vi "Post Upload.vi"() -> ()   [LabVIEW 2012]
uses:
  <vilib>/LVH/i3 Twitter/i3-twitter.lvlib
  <vilib>/LVH/i3 Twitter/SubVIs/Twitter Open - Desktop.vi
  <vilib>/LVH/i3 Twitter/Tweets with Media/Post Media Tweet - From File.vi
panel:
  out "resulting string":string
  out "file names":string[](array[string])
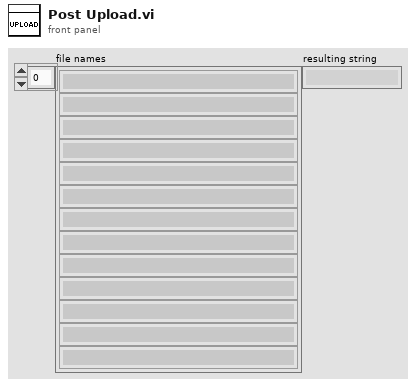
[diagram p1: front panel]
types:
  T1 = typedef "i3-twitter.lvlib/Twitter Handle.ctl" = cluster{"OAuth Credentials":T2, "since ID":string, "max ID":string, "Screen Name":string}
  T2 = typedef "i3-oauth.lvlib/OAuth Handle.ctl" = cluster{"Signature Method":T3, "Version":string, "Client":T4, "Access":T4}
  T3 = typedef "i3-oauth.lvlib/Signature Method.ctl" = enum16{"HMAC-MD5", "HMAC-SHA1", "HMAC-SHA224", "HMAC-SHA256", "HMAC-SHA384", "HMAC-SHA512"}
  T4 = typedef "i3-oauth.lvlib/Credentials.ctl" = cluster{"Token":string, "Secret":string}
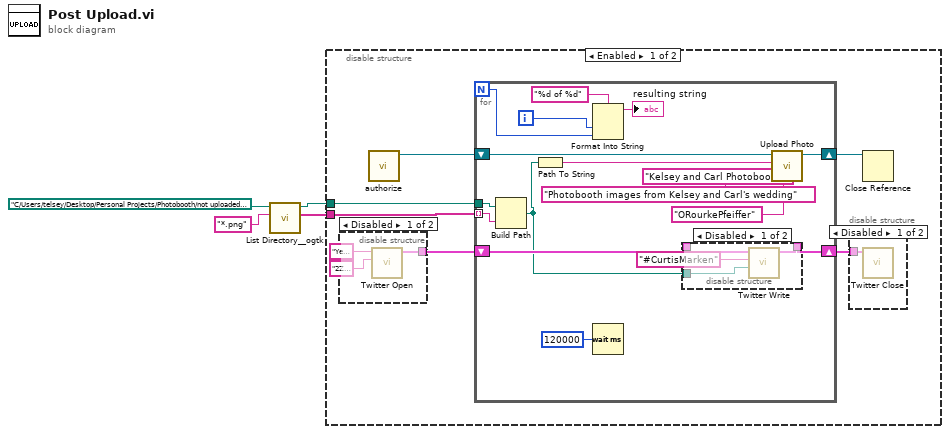
[diagram p0: block diagram]
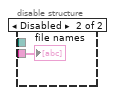
[diagram p5: hidden frame]
diagram:
  n1 = call <userlib>:"List Directory__ogtk.vi"("pattern"="*.png", "directory path"=path "C:/Users/telsey/Desktop/Personal Projects/Photobooth/not uploaded yet") -> ("file names"=w3:string[], "dup directory path"=w1:path)  [unwired: 2 in, 2 out]
  n2 = disable-structure shown="Enabled" {
    disable-tunnel: w3 -> [w6 w35]
    disable-tunnel: w1 -> [w5 _]
    frame Enabled {
      n3 = disable-structure shown="Disabled" {
        disable-tunnel: [w12 _] -> w10
        frame Disabled {
          n4 = call-poly <vilib>:"Twitter Open.vi"("Consumer Secret"="2ZDmzpqyNpiByDQQhohs8dSN9LtSH3nAod3QldeU", "Consumer Key"="Ye1QTjAaMzT6uHrDUqJR2w") -> ("Twitter Handle Out"=w12:T1)  [unwired: 7 in, 2 out]
        }
        frame Enabled {
        }
      }
      n5 = call "authorize.vi"() -> ("Flickr Ref out"=w9:refnum<k24>)  [unwired: 11 in]
      n6 = for {
        N -> [w16]
        shift-right: [w29] -> w7
        shift-left: w10 -> [w30]
        shift-right: [w24] -> w8
        shift-left: w9 -> [w28]
        tunnel: w6 -> [w23] mode=indexing
        tunnel: w5 -> [w22]
        i -> [w17]
        n7 = Build Path(base path=w22, name or relative path=w23) -> (appended path=w21:path)
        n8 = Path To String(path=w21) -> (string=w20:string)
        n9 = Format Into String(format string="%d of %d", w17, w16) -> (resulting string=→"resulting string":string)  [unwired: 2 in, 1 out]
        n10 = Wait (ms)(milliseconds to wait=u32 120000) -> ()  [unwired: 1 out]
        n11 = disable-structure shown="Disabled" {
          disable-tunnel: w30 -> [w34 _]
          disable-tunnel: [w32 _] -> w29
          disable-tunnel: w21 -> [w31 _]
          frame Disabled {
            n12 = call-poly <vilib>:"Twitter Write.vi"("Picture File (PNG, JPG, GIF)"=w31, "Tweet"="#CurtisMarken", "Twitter Handle In"=w34) -> ("Twitter Handle Out"=w32:T1)  [unwired: 7 in, 1 out]
          }
          frame Enabled {
          }
        }
        n13 = call "Upload Photo.vi"("Photo tags"="ORourkePfeiffer", "Description"="Photobooth images from Kelsey and Carl's wedding", "Photoset Name"="Kelsey and Carl Photobooth", "Image Path"=w20, "Flickr Ref"=w28) -> ("Flickr Ref out"=w24:refnum<k24>)  [unwired: 6 in]
      }
      n14 = disable-structure shown="Disabled" {
        disable-tunnel: w7 -> [w11 _]
        frame Disabled {
          n15 = call <vilib>:"Twitter Close.vi"("Twitter Handle In"=w11) -> ()  [unwired: 10 in, 1 out]
        }
        frame Enabled {
        }
      }
      n16 = Close Reference(reference=w8) -> ()  [unwired: 1 in, 1 out]
    }
    frame Disabled {
      "file names" <- w35
    }
  }
